vi "DHE_GetFPAname.vi"() -> (7 "DHE_FPAname":string)   [LabVIEW 2016]
uses:
  private/vis/DHE_GBLDriverVariables.vi
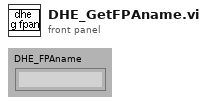
[diagram p1: front panel]
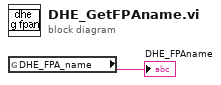
[diagram p0: block diagram]
diagram:
  n1 = global read "DHE_GBLDriverVariables.vi" "DHE_FPA_name"() -> (→"DHE_FPAname":string)
